vi "SSC Digital PPMU Source Voltage.vi"(0 "Digital SSC in":T1[](array[typedef]), 5 "Voltage Level (V)":dbl format="%#_6p", 7 "Current Limit Range (A)":dbl format="%#_6p", 11 "error in":errorcluster) -> (4 "Digital SSC out":T1[](array[typedef]), 15 "error out":errorcluster)   [LabVIEW 2020]
doc: "Starts sourcing voltage from the PPMU on the specified pin(s) and pin group(s). This VI automatically selects the PPMU function. Changes to PPMU source settings do not take effect until you call this VI."
uses:
  SSC Digital.ctl
  <instrlib>/niDigital/niDigital.llb/niDigital Output Function.ctl
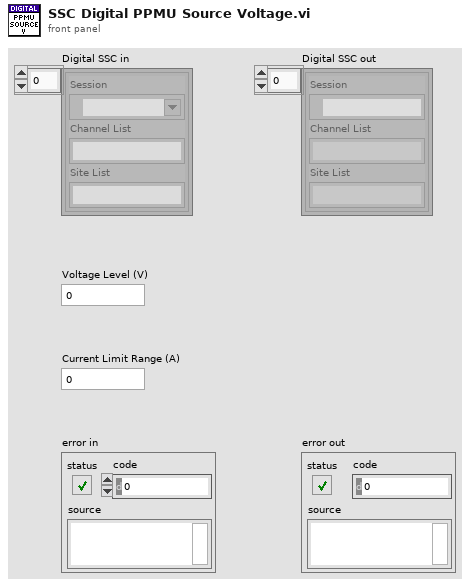
[diagram p1: front panel]
types:
  T1 = typedef "SSC Digital.ctl" = cluster{"Session":refnum<k15>, "Channel List":string, "Site List":string}
  T2 = typedef "niDigital Output Function.ctl" = i32
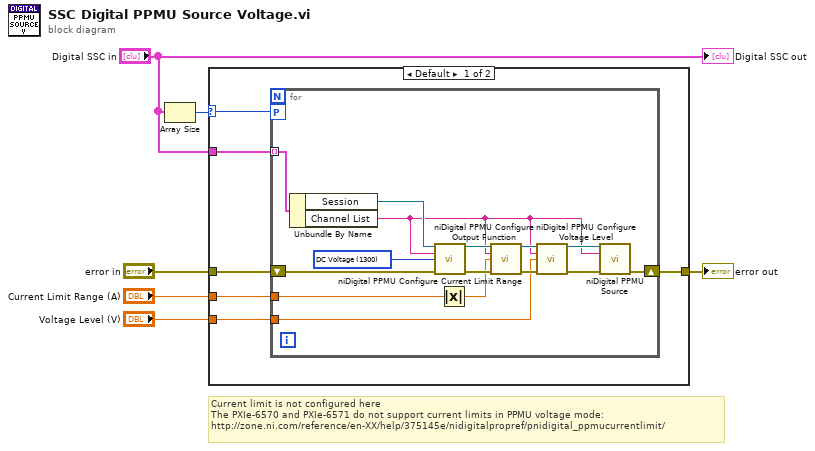
[diagram p0: block diagram]
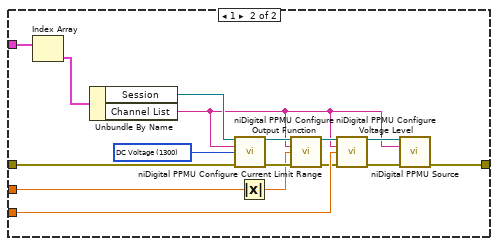
[diagram p2: hidden frame]
diagram:
  # "Current limit is not configured here\nThe PXIe-6570 and PXIe-6571 do not support current limits in PPMU voltage mode:\nhttp://zone.ni.com/reference/en-XX/help/375145e/nidigitalpropref/pnidigital_ppmucurrentlimit/"
  n1 = Array Size(array="Digital SSC in") -> (size(s)=w2:i32)
  n2 = case shown="Default" w2 {
    selector: w2 -> [w8 _]
    tunnel: "error in" -> [w12 w43]
    tunnel: "Current Limit Range (A)" -> [w11 w42]
    tunnel: "Voltage Level (V)" -> [w10 w41]
    tunnel: [w9 w40] -> w3
    tunnel: "Digital SSC in" -> [w7 w39]
    frame Default {
      n3 = for {
        tunnel: w11 -> [w18]
        tunnel: w10 -> [w17]
        workers-P: w8 -> [_]
        tunnel: w7 -> [w15] mode=indexing
        shift-right: [w19] -> w9
        shift-left: w12 -> [w22]
        w23 = T2 1300 items=["DC Voltage"=1300, "DC Current"=1301] ("output function")
        n4 = Unbundle By Name(w15) -> ("Session"=w14:refnum<k15>, "Channel List"=w13:string)
        n5 = call <instrlib>:"niDigital PPMU Configure Output Function.vi"("instrument handle"=w14, "channel list"=w13, "output function"=w23, "error in"=w22) -> ("instrument handle out"=w24:refnum<k15>, "error out"=w27:errorcluster)  [unwired: 10 in]
        n6 = Absolute Value(x=w18) -> (abs(x)=w16:dbl)
        n7 = call <instrlib>:"niDigital PPMU Configure Current Limit Range.vi"("instrument handle"=w24, "channel list"=w13, "current limit range (A)"=w16, "error in"=w27) -> ("instrument handle out"=w25:refnum<k15>, "error out"=w26:errorcluster)  [unwired: 10 in]
        n8 = call <instrlib>:"niDigital PPMU Configure Voltage Level.vi"("instrument handle"=w25, "channel list"=w13, "voltage level (V)"=w17, "error in"=w26) -> ("instrument handle out"=w20:refnum<k15>, "error out"=w21:errorcluster)  [unwired: 10 in]
        n9 = call <instrlib>:"niDigital PPMU Source.vi"("instrument handle"=w20, "channel list"=w13, "error in"=w21) -> ("error out"=w19:errorcluster)  [unwired: 11 in, 1 out]
      }
    }
    frame 1 {
      w34 = T2 1300 items=["DC Voltage"=1300, "DC Current"=1301] ("output function")
      n10 = Index Array(array=w39) -> (element=w28:T1)  [unwired: 1 in]
      n11 = Unbundle By Name(w28) -> ("Session"=w30:refnum<k15>, "Channel List"=w29:string)
      n12 = call <instrlib>:"niDigital PPMU Configure Output Function.vi"("instrument handle"=w30, "channel list"=w29, "output function"=w34, "error in"=w43) -> ("instrument handle out"=w35:refnum<k15>, "error out"=w38:errorcluster)  [unwired: 10 in]
      n13 = Absolute Value(x=w42) -> (abs(x)=w31:dbl)
      n14 = call <instrlib>:"niDigital PPMU Configure Current Limit Range.vi"("instrument handle"=w35, "channel list"=w29, "current limit range (A)"=w31, "error in"=w38) -> ("instrument handle out"=w36:refnum<k15>, "error out"=w37:errorcluster)  [unwired: 10 in]
      n15 = call <instrlib>:"niDigital PPMU Configure Voltage Level.vi"("instrument handle"=w36, "channel list"=w29, "voltage level (V)"=w41, "error in"=w37) -> ("instrument handle out"=w32:refnum<k15>, "error out"=w33:errorcluster)  [unwired: 10 in]
      n16 = call <instrlib>:"niDigital PPMU Source.vi"("instrument handle"=w32, "channel list"=w29, "error in"=w33) -> ("error out"=w40:errorcluster)  [unwired: 11 in, 1 out]
    }
  }
  "error out" <- w3
  "Digital SSC out" <- "Digital SSC in"
